vi "arrange.vi"(1 "Input Array":i32[][](array[numeric])) -> (0 "Ordered Coordinates":i32[][](array[numeric]))   [LabVIEW 2014]
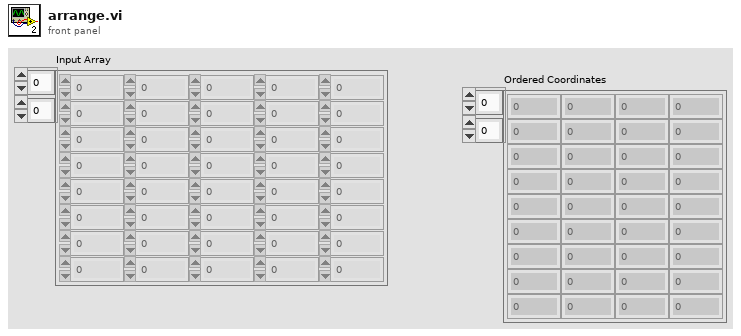
[diagram p1: front panel]
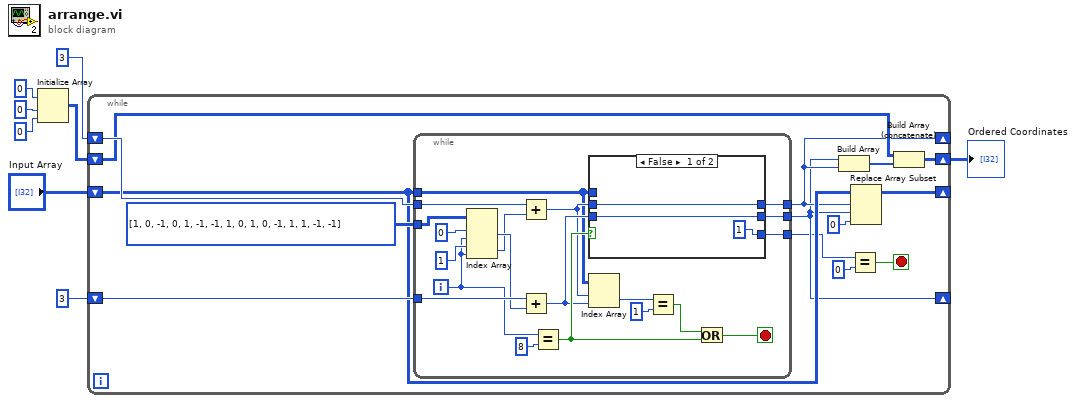
[diagram p0: block diagram]
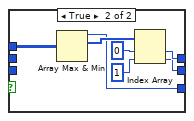
[diagram p2: hidden frame]
diagram:
  n1 = Initialize Array(0, 0, 0) -> (w2:i32[][])
  n2 = while {
    shift-right: [w12] -> _
    shift-left: 3 -> [w22]
    shift-right: [w13] -> _
    shift-left: 3 -> [w21]
    shift-right: [w17] -> w1
    shift-left: w2 -> [w19]
    shift-right: [w15] -> _
    shift-left: "Input Array" -> [w16]
    stop <- w9 stop-if-true
    n3 = while {
      tunnel: w16 -> [w24]
      tunnel: w22 -> [w42]
      tunnel: w21 -> [w39]
      tunnel: [w25] -> w13
      tunnel: [w27] -> w12
      tunnel: i32[][] [[1, 0, -1, 0, 1, -1, -1, 1], [0, 1, 0, -1, 1, 1, -1, -1]] -> [w38]
      tunnel: [w23] -> w10
      i -> [w32]
      stop <- w30 stop-if-true
      n4 = Index Array(array=w38, index (row) #1=0, index (col) #1=w32, index (row) #2=1, index (col) #2=w32) -> (element #1=w35:i32, element #2=w34:i32)
      n5 = Add(x=w39, y=w34) -> (x+y=w26:i32)
      n6 = Add(x=w42, y=w35) -> (x+y=w28:i32)
      n7 = Equal?(x=w32, y=8) -> (x = y?=w29:bool)
      n8 = case shown="False" w29 {
        tunnel: w28 -> [w45 _]
        tunnel: [w45 w49] -> w27
        tunnel: w26 -> [w44 _]
        tunnel: [w44 w50] -> w25
        tunnel: w24 -> [_ w52]
        tunnel: [1 w46] -> w23
        frame False {
        }
        frame True {
          n9 = Array Max & Min(array=w52) -> (max value=w46:i32, max index (indices)=w51:i32[])  [unwired: 2 out]
          n10 = Index Array(array=w51, index #1=0, index #2=1) -> (element #1=w50:i32, element #2=w49:i32)
        }
      }
      n11 = Index Array(array=w24, index (row)=w26, index (col)=w28) -> (element=w40:i32)
      n12 = Equal?(x=w40, y=1) -> (x = y?=w33:bool)
      n13 = Or(x=w33, y=w29) -> (x .or. y?=w30:bool)
    }
    n14 = Build Array(w12, w13) -> (w18:i32[])
    n15 = Equal?(x=w10, y=0) -> (x = y?=w9:bool)
    n16 = Replace Array Subset(array=w16, new element=0, index (row)=w13, index (col)=w12) -> (w15:i32[][])
    n17 = Build Array (concatenate)(w19, w18) -> (w17:i32[][])
  }
  "Ordered Coordinates" <- w1
